vi "sub_new x y amplitude.vi"(7 "Global Rectangle":i32[](array[numeric]), 8 "Line":u16, 9 "Pixel/Line":u16, 10 "y amp.":dbl, 11 "x amp.":dbl) -> (0 "y offset new":i16, 1 "x offset new":i16, 2 "y amp. new":dbl, 3 "x amp. new":dbl)   [LabVIEW 2015]
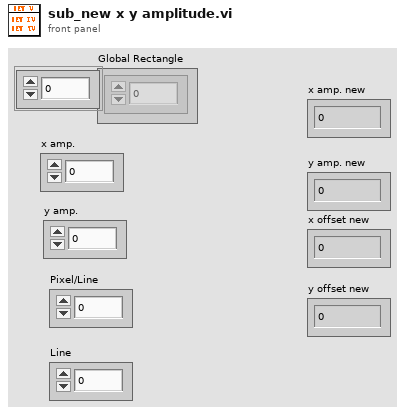
[diagram p1: front panel]
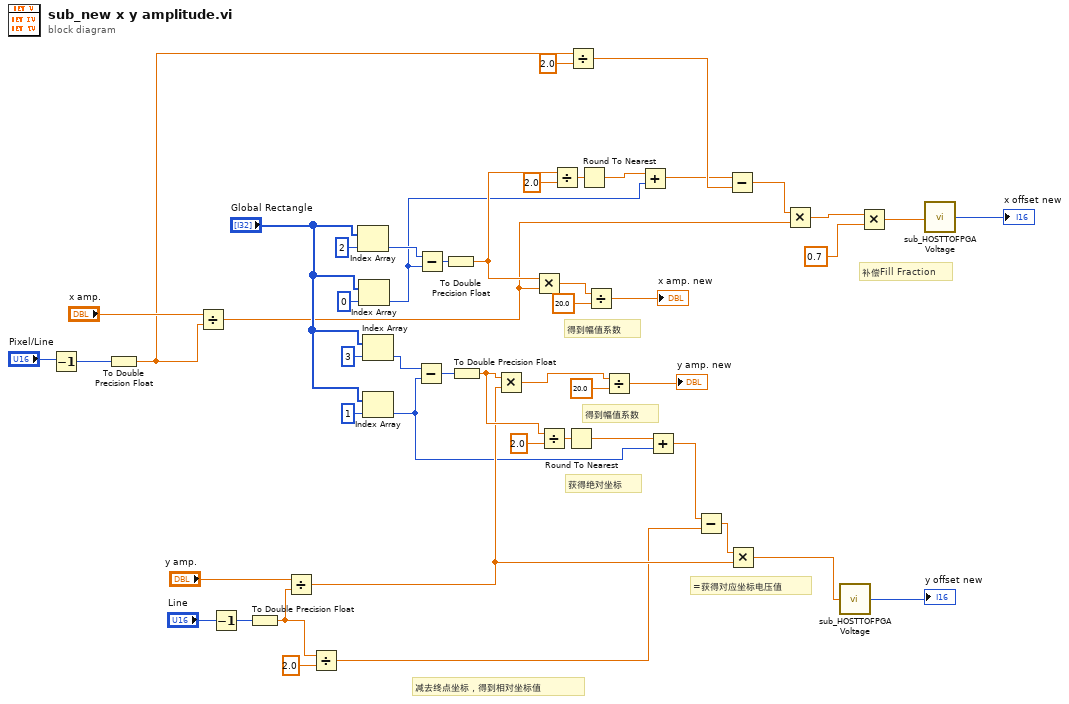
[diagram p0: block diagram]
diagram:
  # "补偿Fill Fraction"
  # "获得绝对坐标"
  # "减去终点坐标，得到相对坐标值"
  # "=获得对应坐标电压值"
  # "得到幅值系数"
  # "得到幅值系数"
  n1 = Decrement(x="Pixel/Line") -> (x-1=w4:u16)
  n2 = To Double Precision Float(number=w4) -> (double precision float=w13:dbl)
  n3 = Divide(x="x amp.", y=w13) -> (x/y=w35:dbl)
  n4 = Decrement(x="Line") -> (x-1=w3:u16)
  n5 = To Double Precision Float(number=w3) -> (double precision float=w5:dbl)
  n6 = Divide(x="y amp.", y=w5) -> (x/y=w30:dbl)
  n7 = Divide(x=w5, y=2.0) -> (x/y=w10:dbl)
  n8 = Index Array(array="Global Rectangle", index=2 ("索引")) -> (element=w42:i32)
  n9 = Index Array(array="Global Rectangle", index=0 ("索引")) -> (element=w6:i32)
  n10 = Index Array(array="Global Rectangle", index=3 ("索引")) -> (element=w46:i32)
  n11 = Index Array(array="Global Rectangle", index=1 ("索引")) -> (element=w8:i32)
  n12 = Subtract(x=w46, y=w8) -> (x-y=w49:i32)
  n13 = Subtract(x=w42, y=w6) -> (x-y=w48:i32)
  n14 = To Double Precision Float(number=w48) -> (double precision float=w39:dbl)
  n15 = To Double Precision Float(number=w49) -> (double precision float=w31:dbl)
  n16 = Multiply(x=w31, y=w30) -> (x*y=w18:dbl)
  n17 = Multiply(x=w39, y=w35) -> (x*y=w22:dbl)
  n18 = Divide(x=w31, y=2.0) -> (x/y=w33:dbl)
  n19 = Divide(x=w39, y=2.0) -> (x/y=w37:dbl)
  n20 = Round To Nearest(number=w33) -> (nearest integer value=w34:dbl)
  n21 = Divide(x=w13, y=2.0) -> (x/y=w12:dbl)
  n22 = Round To Nearest(number=w37) -> (nearest integer value=w36:dbl)
  n23 = Divide(x=w22, y=20.0) -> (x/y=→"x amp. new":dbl)
  n24 = Divide(x=w18, y=20.0) -> (x/y=→"y amp. new":dbl)
  n25 = Add(x=w36, y=w6) -> (x+y=w7:dbl)
  n26 = Add(x=w34, y=w8) -> (x+y=w9:dbl)
  n27 = Subtract(x=w9, y=w10) -> (x-y=w11:dbl)
  n28 = Subtract(x=w7, y=w12) -> (x-y=w15:dbl)
  n29 = Multiply(x=w11, y=w30) -> (x*y=w26:dbl)
  n30 = Multiply(x=w15, y=w35) -> (x*y=w16:dbl)
  n31 = call "sub_HOSTTOFPGA Voltage.vi"("Input"=w26) -> ("Output"=→"y offset new":i16)
  n32 = Multiply(x=w16, y=0.7 ("x")) -> (x*y=w2:dbl)
  n33 = call "sub_HOSTTOFPGA Voltage.vi"("Input"=w2) -> ("Output"=→"x offset new":i16)
